vi "MGI Separate String.vi"(9 "Separators":string[](array[string]), 11 "String":string) -> (3 "Separated String":string[](array[string]))   [LabVIEW 2020]
doc: "Separates <b>String</b> by breaking it up into separate elements in <b>Separated String</b> at the <b>separators</b>, but without taking out the separators. For example, the string 1-2/3 with separators - and / would output the array {\"1-\" \"2/\" \"3\"}.\nNote: Separators must be single characters.\n\nAuthored by Hope Harrison\nsupport@mooregoodideas.com\nwww.mooregoodideas.com\n\nCopyright (c) 2010, Moore Good Ideas, Inc.\n\nAll rights reserved.\n\nRedistribution and use in source and binary forms, with or without modification, are permitted provided that the following conditions are met:\n\n * Redistributions of source code must retain the above copyright notice, this list of conditions and the following disclaimer.\n * Redistributions in binary form must reproduce the above copyright notice, this list of conditions and the following disclaimer in the documentation and/or other materials provided with the distribution.\n * Neither the name of Moore Good Ideas, Inc. nor the names of its contributors may be used to endorse or promote products derived from this software without specific prior written permission.\n\nTHIS SOFTWARE IS PROVIDED BY THE COPYRIGHT HOLDERS AND CONTRIBUTORS \"AS IS\" AND ANY EXPRESS OR IMPLIED WARRANTIES, INCLUDING, BUT NOT LIMITED TO, THE IMPLIED WARRANTIES OF MERCHANTABILITY AND FITNESS FOR A PARTICULAR PURPOSE ARE DISCLAIMED. IN NO EVENT SHALL THE COPYRIGHT OWNER OR CONTRIBUTORS BE LIABLE FOR ANY DIRECT, INDIRECT, INCIDENTAL, SPECIAL, EXEMPLARY, OR CONSEQUENTIAL DAMAGES (INCLUDING, BUT NOT LIMITED TO, PROCUREMENT OF SUBSTITUTE GOODS OR SERVICES; LOSS OF USE, DATA, OR PROFITS; OR BUSINESS INTERRUPTION) HOWEVER CAUSED AND ON ANY THEORY OF LIABILITY, WHETHER IN CONTRACT, STRICT LIABILITY, OR TORT (INCLUDING NEGLIGENCE OR OTHERWISE) ARISING IN ANY WAY OUT OF THE USE OF THIS SOFTWARE, EVEN IF ADVISED OF THE POSSIBILITY OF SUCH DAMAGE."
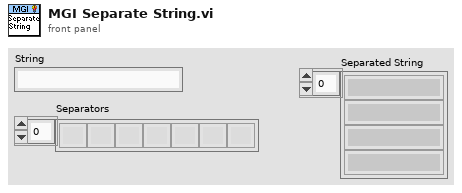
[diagram p1: front panel]
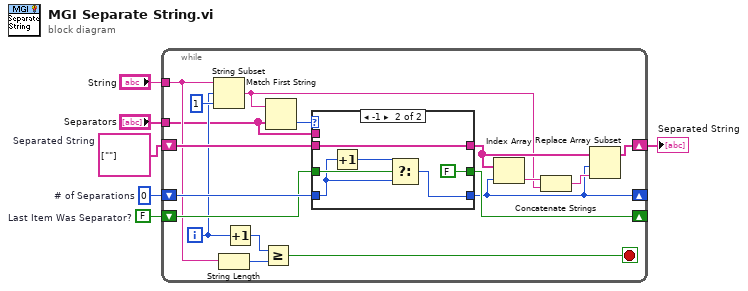
[diagram p0: block diagram]
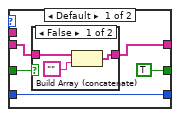
[diagram p2: hidden frame]
diagram:
  w2 = FALSE  # Last Item Was Separator?
  w4 = string[] [""]  # Separated String
  w3 = 0  # # of Separations
  n1 = while {
    tunnel: "String" -> [w13]
    tunnel: "Separators" -> [w8]
    shift-right: [w14] -> _
    shift-left: w3 -> [w22]
    shift-right: [w15] -> w1
    shift-left: w4 -> [w23]
    shift-right: [w18] -> _
    shift-left: w2 -> [w21]
    i -> [w12]
    stop <- w10 stop-if-true
    n2 = String Subset(string=w13, offset (0)=w12, length (rest)=1 ("length (rest)")) -> (substring=w7:string)
    n3 = String Length(string=w13) -> (length=w9:i32)
    n4 = Increment(x=w12) -> (x+1=w11:i32)
    n5 = Greater Or Equal?(x=w11, y=w9) -> (x >= y?=w10:bool)
    n6 = Match First String(2:w8, 3:w7) -> (0:w19:i32)  [unwired: 1 out]
    n7 = case shown="-1" w19 {
      tunnel: w23 -> [w27 w36]
      tunnel: w22 -> [w29 w37]
      tunnel: w8 -> [_ _]
      tunnel: w21 -> [w26 w39]
      tunnel: [w25 w36] -> w17
      tunnel: [w29 w35] -> w14
      tunnel: [TRUE ("Last Item Was Separator?") FALSE ("Last Item Was Separator?")] -> w18
      frame Default {
        n8 = case shown="False" w26 {
          tunnel: w27 -> [w32 w33]
          tunnel: [w31 w33] -> w25
          frame False {
            n9 = Build Array (concatenate)(w32, "") -> (w31:string[])
          }
          frame True {
          }
        }
      }
      frame -1 {
        n10 = Increment(x=w37) -> (x+1=w38:i32)
        n11 = Select(t=w38, s=w39, f=w37) -> (s? t:f=w35:i32)
      }
    }
    n12 = Index Array(array=w17, index=w14) -> (element=w16:string)
    n13 = Concatenate Strings(w16, w7) -> (w20:string)
    n14 = Replace Array Subset(array=w17, new element=w20, index=w14) -> (w15:string[])
  }
  "Separated String" <- w1
